vi "Create Initial Files.vi"(8 "error in (no error)":errorcluster, 11 "Setup File in":refnum<class "Setup File.lvclass">) -> (0 "error out":errorcluster, 3 "Setup File out":refnum<class "Setup File.lvclass">)   [LabVIEW 2012, in "Setup File.lvclass"]
uses:
  Setup File.lvclass
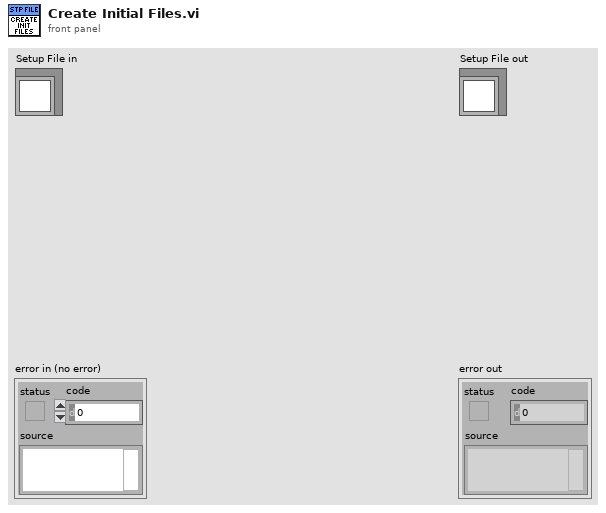
[diagram p1: front panel]
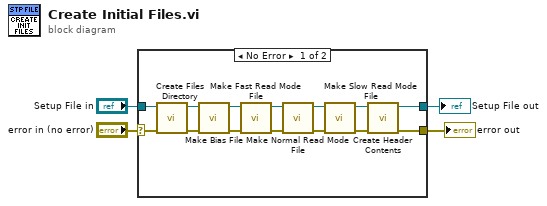
[diagram p0: block diagram]
diagram:
  n1 = case shown="No Error" "error in (no error)" {
    selector: "error in (no error)" -> [w17 w20]
    tunnel: [w5 w20] -> w2
    tunnel: [w6 w19] -> w1
    tunnel: "Setup File in" -> [w18 w19]
    frame No Error {
      n2 = call "Create Files Directory.vi"("error in (no error)"=w17, "Setup File in"=w18) -> ("error out"=w15:errorcluster, "Setup File out"=w16:refnum<class "Setup File.lvclass">)  [unwired: 8 in]
      n3 = call "Make Bias File.vi"("error in (no error)"=w15, "Setup File in"=w16) -> ("error out"=w14:errorcluster, "Setup File out"=w9:refnum<class "Setup File.lvclass">)  [unwired: 8 in]
      n4 = call "Make Fast Read Mode File.vi"("error in (no error)"=w14, "Setup File in"=w9) -> ("error out"=w13:errorcluster, "Setup File out"=w10:refnum<class "Setup File.lvclass">)  [unwired: 8 in]
      n5 = call "Make Normal Read Mode File.vi"("error in (no error)"=w13, "Setup File in"=w10) -> ("error out"=w12:errorcluster, "Setup File out"=w11:refnum<class "Setup File.lvclass">)  [unwired: 8 in]
      n6 = call "Make Slow Read Mode File.vi"("error in (no error)"=w12, "Setup File in"=w11) -> ("error out"=w8:errorcluster, "Setup File out"=w7:refnum<class "Setup File.lvclass">)  [unwired: 8 in]
      n7 = call "Create Header Contents.vi"("error in (no error)"=w8, "Setup File in"=w7) -> ("error out"=w5:errorcluster, "Setup File out"=w6:refnum<class "Setup File.lvclass">)  [unwired: 8 in]
    }
    frame Error {
    }
  }
  "error out" <- w2
  "Setup File out" <- w1
